vi "Toggle Output with Preset.vi"(7 "reset value":bool, 9 "reset":bool, 10 "toggle":bool) -> (2 "output":bool)   [LabVIEW 2023, in "niUSRP Rx Core v1 FPGA.lvclass"]
doc: "<b>Pipeline Delay = 0</b>"
uses:
  <instrlib>/niUSRP/Reference FPGA/Rx Core/niUSRP Rx Core v1 FPGA.lvclass
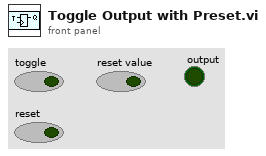
[diagram p1: front panel]
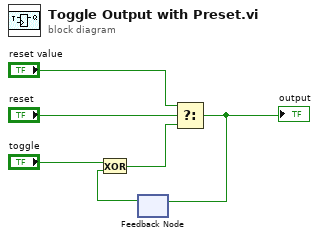
[diagram p0: block diagram]
diagram:
  n1 = feedback #1() -> (w5:bool)  [unwired: 1 in]
  n2 = Exclusive Or(1:w5, 2:"toggle") -> (0:w1:bool)
  n3 = Select(t="reset value", s="reset", f=w1) -> (s? t:f=w2:bool)
  "output" <- w2
  n4 = feedback-in #1(w2) -> ()
